vi "Evaluate.vi"(8 "error in (no error)":errorcluster, 11 "Environment.LogFile in":refnum<class "Environment.LogFile.lvclass">) -> (0 "error out":errorcluster, 3 "Environment.LogFile out":refnum<class "Environment.LogFile.lvclass">)   [LabVIEW 2018, in "Environment.LogFile.lvclass"]
uses:
  Environment.LogFile.lvclass
  C:/Users/Colin/Documents/software_projects/labview/unit_testing_fw/Environment/Environment.lvclass
  unit_testing_fw/Environment/Environment.lvclass/Environment.ctl
  Environment.LogFile.lvclass/Environment.LogFile.ctl
  unit_testing_fw/Environment/Environment.lvclass
  <vilib>/addons/_JKI Toolkits/Caraya/classes/Assert/Assert.lvclass
  <vilib>/addons/_JKI Toolkits/Caraya/classes/Test/Test.lvclass
panel:
  # "Connector Pane"
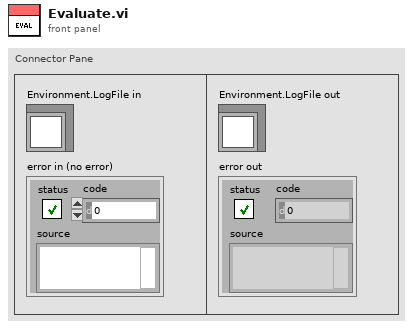
[diagram p1: front panel]
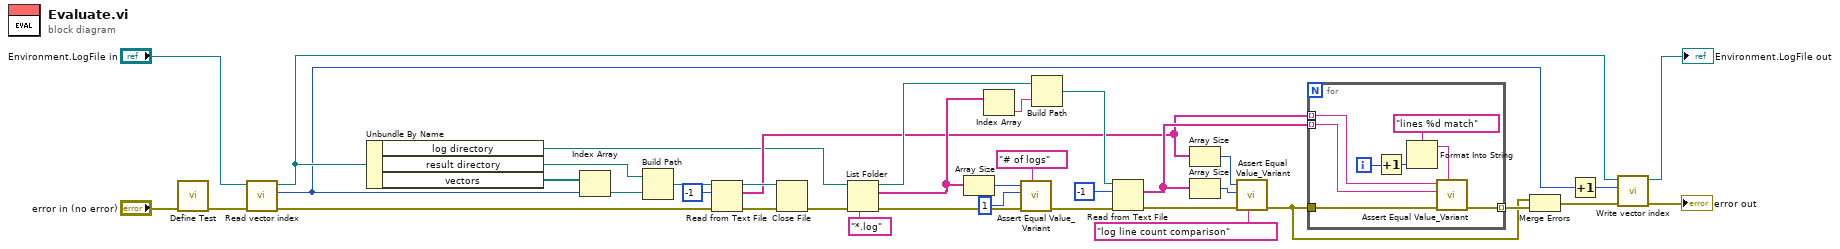
[diagram p0: block diagram]
diagram:
  n1 = call <vilib>:"Define Test.vi"("error in (no error)"="error in (no error)") -> ("error out"=w1:errorcluster)  [unwired: 9 in, 1 out]
  n2 = call "Read vector index.vi"("error in (no error)"=w1, "Environment in"="Environment.LogFile in") -> ("error out"=w29:errorcluster, "vector index"=w2:i32, "Environment out"=w36:refnum<class "Environment.LogFile.lvclass">)  [unwired: 7 in]
  n3 = Unbundle By Name(w36) -> ("log directory"=w3:path, "result directory"=w34:path, "vectors"=w35:path[])
  n4 = Index Array(array=w35, index=w2) -> (element=w33:path)
  n5 = Build Path(base path=w34, name or relative path=w33) -> (appended path=w32:path)
  n6 = Read from Text File(file (use dialog)=w32, count=-1, error in=w29) -> (refnum out=w30:refnum<file>, text=w10:string[], error out=w31:errorcluster)  [unwired: 1 in, 1 out]
  n7 = Close File(refnum=w30, error in=w31) -> (error out=w28:errorcluster)  [unwired: 1 out]
  n8 = List Folder(path=w3, pattern="*.log", error in=w28) -> (path out=w20:path, filenames=w22:string[], error out=w23:errorcluster)  [unwired: 1 in, 1 out]
  n9 = Array Size(array=w22) -> (size(s)=w26:i32)
  n10 = Index Array(array=w22) -> (element=w21:string)  [unwired: 1 in]
  n11 = call <vilib>:"Assert Equal Value_Variant.vi"("Label"="# of logs", "error in (no error)"=w23, "Y"=1 ("size(s)"), "X"=w26) -> ("error out"=w18:errorcluster)  [unwired: 6 in, 1 out]
  n12 = Build Path(base path=w20, name or relative path=w21) -> (appended path=w19:path)
  n13 = Read from Text File(file (use dialog)=w19, count=-1, error in=w18) -> (text=w11:string[], error out=w12:errorcluster)  [unwired: 1 in, 2 out]
  n14 = Array Size(array=w10) -> (size(s)=w15:i32)
  n15 = Array Size(array=w11) -> (size(s)=w14:i32)
  n16 = call <vilib>:"Assert Equal Value_Variant.vi"("Label"="log line count comparison", "error in (no error)"=w12, "Y"=w14, "X"=w15) -> ("error out"=w8:errorcluster)  [unwired: 6 in, 1 out]
  n17 = for {
    tunnel: w10 -> [w46] mode=indexing
    tunnel: w11 -> [w45] mode=indexing
    tunnel: w8 -> [w40]
    tunnel: [w39] -> w9 mode=indexing
    i -> [w44]
    n18 = Increment(x=w44) -> (x+1=w42:i32)
    n19 = Format Into String(format string="lines %d match" ("Label"), w42) -> (resulting string=w41:string)  [unwired: 2 in, 1 out]
    n20 = call <vilib>:"Assert Equal Value_Variant.vi"("Label"=w41, "error in (no error)"=w40, "Y"=w45, "X"=w46) -> ("error out"=w39:errorcluster)  [unwired: 6 in, 1 out]
  }
  n21 = Merge Errors(w8, w9) -> (w5:errorcluster)
  n22 = Increment(x=w2) -> (x+1=w6:i32)
  n23 = call "Write vector index.vi"("error in (no error)"=w5, "vector index"=w6, "Environment in"=w36) -> ("error out"=→"error out":errorcluster, "Environment out"=→"Environment.LogFile out":refnum<class "Environment.LogFile.lvclass">)  [unwired: 7 in]
